vi "SplitString.vi"(11 "Command":string) -> (3 "Array":string[](array[string]))   [LabVIEW 2018]
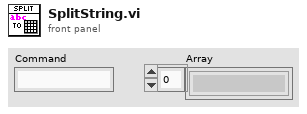
[diagram p1: front panel]
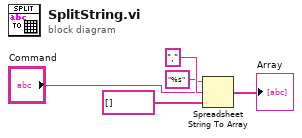
[diagram p0: block diagram]
diagram:
  n1 = Spreadsheet String To Array(delimiter (Tab)=",", format string="%s", spreadsheet string="Command", array type (2D Dbl)=string[] [] ("Array")) -> (array=→"Array":string[])
